vi "Phase Test.vi"() -> ()   [LabVIEW 2019]
uses:
  <vilib>/Analysis/NI_AALPro.lvlib
panel:
  in  "Delay":dbl=1.08e-07 format="%#_6p"
  in  "X":dbl[](array[numeric])=[0.761, 0.7957, 0.7991, 0.75425, 0.661, 0.1077, -0.6861]
  out "XY Graph 2":cluster{"F":dbl[], "Y":dbl[]}[](graph)=[{"F"=[8267.2, 49603.2, 99206.3, 496032.0, 992063.0, 0.0, 5208330.0], "Y"=[0.0128, -0.0115, -0.0474, -0.2805, -0.5301, -0.79678, 0.4875]}, {"F"=[8267.2, 49603.2, 99206.3, 496032.0, 992063.0, 0.0, 5208330.0], "Y"=[0.01706897838906497, 0.015284669929272238, 0.006462002578888259, -0.01564615301365522, -0.002322392747441329, -0.79678, -0.18783402492636733]}]
  out "XY Graph":cluster{"F":dbl[], dbl[]}[](graph)=[{"F"=[8267.2, 49603.2, 99206.3, 496032.0, 992063.0, 0.0, 5208330.0], [0.016818387799899793, -0.014451677005748863, -0.059247309681085124, -0.35604360263631074, -0.6759390099955214, -1.4364415730058453, 2.523829281652911]}, {"F"=[8267.2, 49603.2, 99206.3, 496032.0, 992063.0, 0.0, 5208330.0], [0.02242837755362342, 0.019208261516592905, 0.008072499505197096, -0.01944421741289304, -0.002740918132699166, -1.4364415730058453, 6.058118754994718]}]
  in  "Y":dbl[](array[numeric])=[0.0128, -0.0115, -0.0474, -0.2805, -0.5301, -0.79678, 0.4875]
  in  "F":dbl[](array[numeric])=[8267.2, 49603.2, 99206.3, 496032.0, 992063.0, 1984130.0, 5208330.0]
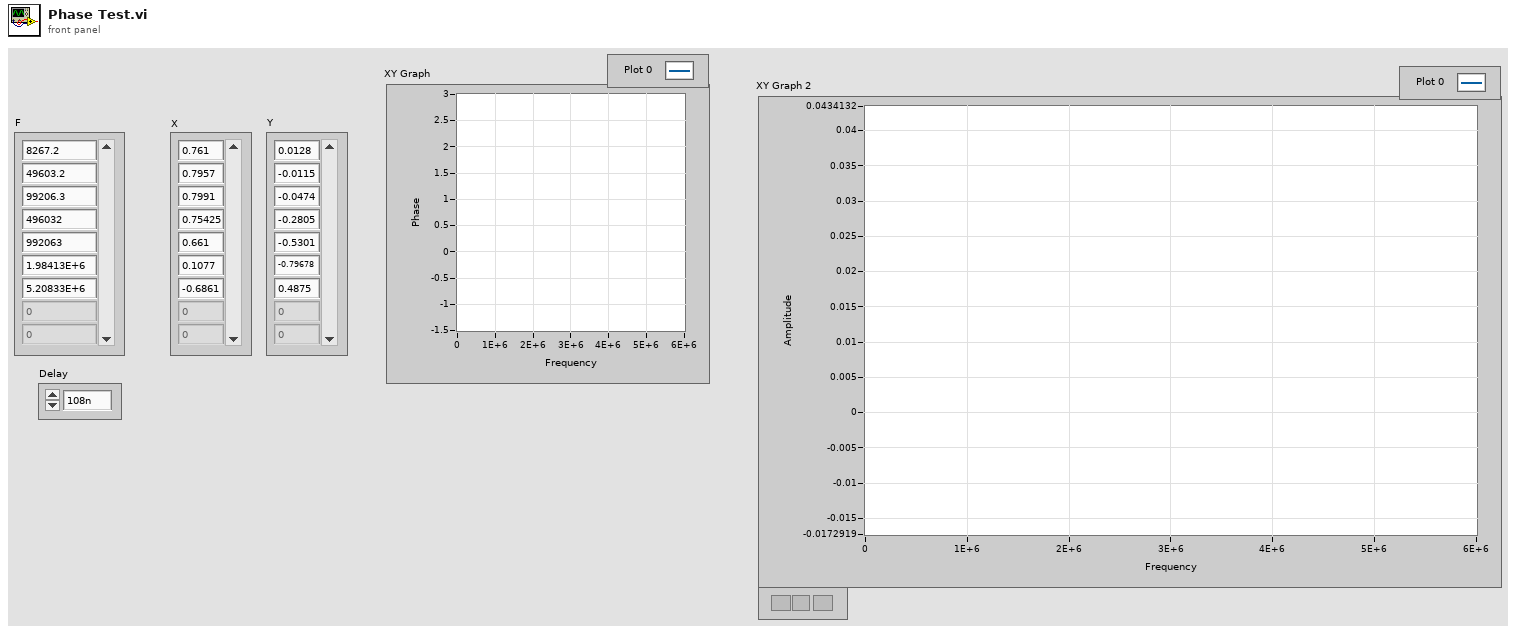
[diagram p1: front panel]
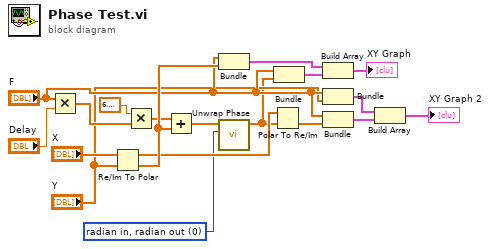
[diagram p0: block diagram]
diagram:
  w4 = 0 items=["radian in, radian out", "radian in, degree out", "degree in, degree out", "degree in, radian out"] ("phase unit")
  n1 = Multiply(x="F", y="Delay") -> (x*y=w16:dbl[])
  n2 = Re/Im To Polar(2:"Y", 3:"X") -> (0:w12:dbl[], 1:w11:dbl[])
  n3 = Multiply(x=6.283185307179586, y=w16) -> (x*y=w3:dbl[])
  n4 = Add(x=w3, y=w12) -> (x+y=w2:dbl[])
  n5 = Bundle("F"="F", w12) -> (w19:cluster{"F":dbl[], dbl[]})  [unwired: 1 in]
  n6 = call <vilib>:"Unwrap Phase.vi"("phase unit"=w4, "Phase"=w2) -> ("Unwrapped Phase"=w1:dbl[])  [unwired: 8 in, 1 out]
  n7 = Polar To Re/Im(2:w1, 3:w11) -> (0:w6:dbl[])  [unwired: 1 out]
  n8 = Bundle("F"="F", "Unwrapped Phase"=w1) -> (w13:cluster{"F":dbl[], "Unwrapped Phase":dbl[]})  [unwired: 1 in]
  n9 = Build Array(w19, w13) -> (→"XY Graph":cluster{"F":dbl[], "Unwrapped Phase":dbl[]}[])
  n10 = Bundle("F"="F", "Y"="Y") -> (w9:cluster{"F":dbl[], "Y":dbl[]})  [unwired: 1 in]
  n11 = Bundle("F"="F", w6) -> (w10:cluster{"F":dbl[], dbl[]})  [unwired: 1 in]
  n12 = Build Array(w9, w10) -> (→"XY Graph 2":cluster{"F":dbl[], "Y":dbl[]}[])
